vi "Format number_123456.vi"(1 "number":i32) -> (0 "String":string)   [LabVIEW 2011]
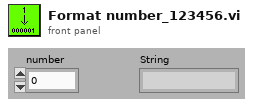
[diagram p1: front panel]
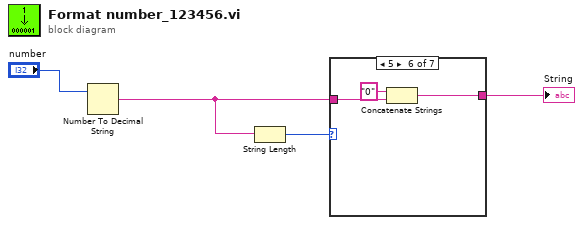
[diagram p0: block diagram]
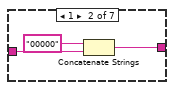
[diagram p3: hidden frame]
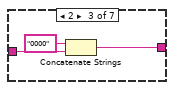
[diagram p4: hidden frame]
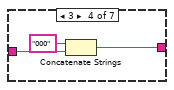
[diagram p5: hidden frame]
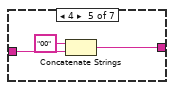
[diagram p6: hidden frame]
diagram:
  n1 = Number To Decimal String(number="number") -> (decimal integer string=w2:string)  [unwired: 1 out]
  n2 = String Length(string=w2) -> (length=w3:i32)
  n3 = case shown="5" w3 {
    tunnel: w2 -> [w5 w8 w11 w14 w17 w20 w21]
    tunnel: [w5 w6 w10 w13 w16 w19 w21] -> w1
    frame 0, Default {
    }
    frame 1 {
      n4 = Concatenate Strings("00000" ("string"), w8) -> (w6:string)
    }
    frame 2 {
      n5 = Concatenate Strings("0000" ("string"), w11) -> (w10:string)
    }
    frame 3 {
      n6 = Concatenate Strings("000" ("string"), w14) -> (w13:string)
    }
    frame 4 {
      n7 = Concatenate Strings("00" ("string"), w17) -> (w16:string)
    }
    frame 5 {
      n8 = Concatenate Strings("0" ("string"), w20) -> (w19:string)
    }
    frame 6 {
    }
  }
  "String" <- w1
